vi "Sequence Update for Spartan 5.0.vi"(8 "error in (no error)":errorcluster, 10 "Old Sequence Record":T1) -> (0 "error out":errorcluster, 2 "New Sequence Record":T1)   [LabVIEW 2011]
uses:
  Sequence Record.ctl
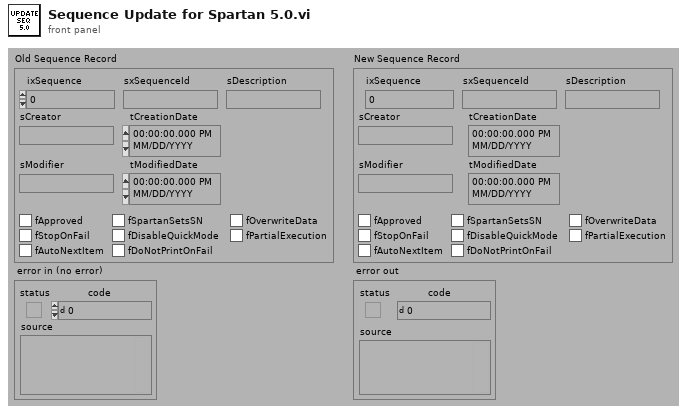
[diagram p1: front panel]
types:
  T1 = typedef "Sequence Record.ctl" = cluster{"ixSequence":i32, "sxSequenceId":string, "sDescription":string, "sCreator":string, "tCreationDate":timestamp, "sModifier":string, "tModifiedDate":timestamp, "fApproved":bool, "fSpartanSetsSN":bool, "fOverwriteData":bool, "fStopOnFail":bool, "fDisableQuickMode":bool, "fPartialExecution":bool, "fAutoNextItem":bool, "fDoNotPrintOnFail":bool}
  T2 = typedef "Sequence Settings.ctl" = cluster{"Overwrite Data":bool, "Note on Repeat":bool, "Stop on First Fail":bool, "Disable QuickMode":bool, "Partial Execution":bool, "Auto Next Item":bool, "NOT USED, DO NOT REMOVE!!!":bool, "Approved":bool}
  T3 = cluster{"Boolean array[0]":bool, "Boolean array[1]":bool}
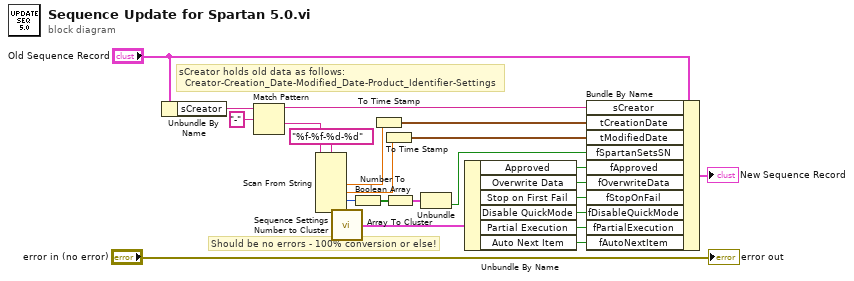
[diagram p0: block diagram]
diagram:
  # "sCreator holds old data as follows:\n  Creator-Creation_Date-Modified_Date-Product_Identifier-Settings"
  # "Should be no errors - 100% conversion or else!"
  n1 = Unbundle By Name("Old Sequence Record") -> ("sCreator"=w19:string)
  n2 = Match Pattern(string=w19, regular expression="-") -> (before substring=w17:string, after substring=w20:string)  [unwired: 3 out]
  n3 = Scan From String(format string="%f-%f-%d-%d", input string=w20) -> (output 1=w4:dbl, output 2=w2:dbl, output 3=w13:i32, output 4=w16:i32)  [unwired: 2 in, 7 out]
  n4 = call "Sequence Settings Number to Cluster.vi"("Sequence Settings"=w16) -> ("Settings"=w12:T2)
  n5 = Number To Boolean Array(number=w13) -> (Boolean array=w15:bool[])
  n6 = To Time Stamp(1:w4) -> (0:w3:timestamp)
  n7 = To Time Stamp(1:w2) -> (0:w1:timestamp)
  n8 = Array To Cluster(array=w15) -> (cluster=w14:T3)
  n9 = Unbundle(w14) -> ("Boolean array[1]"=w5:bool)  [unwired: 1 out]
  n10 = Unbundle By Name(w12) -> ("Approved"=w11:bool, "Overwrite Data"=w10:bool, "Stop on First Fail"=w9:bool, "Disable QuickMode"=w8:bool, "Partial Execution"=w7:bool, "Auto Next Item"=w6:bool)
  n11 = Bundle By Name(cluster="Old Sequence Record", "sCreator"=w17, "tCreationDate"=w3, "tModifiedDate"=w1, "fSpartanSetsSN"=w5, "fApproved"=w11, "fOverwriteData"=w10, "fStopOnFail"=w9, "fDisableQuickMode"=w8, "fPartialExecution"=w7, "fAutoNextItem"=w6) -> (→"New Sequence Record":T1)
  "error out" <- "error in (no error)"
